vi "Replace Sub VI.vi"(8 "error in (no error)":errorcluster, 11 "VI in":refnum<vi>) -> (0 "error out":errorcluster, 3 "VI out":refnum<vi>)   [LabVIEW 2020, in "Responsive Mock Class Generator.lvclass"]
uses:
  Responsive Mock Class Generator.lvclass
  <vilib>/Utility/traverseref.llb/TRef TravTarget.ctl
  <vilib>/Utility/traverseref.llb/VI Scripting - Traverse.lvlib
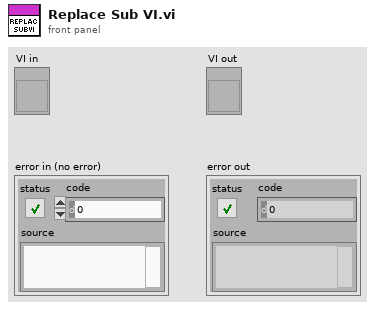
[diagram p1: front panel]
types:
  T1 = typedef "TRef TravTarget.ctl" = enum16{"FP", "BD", "Other"}
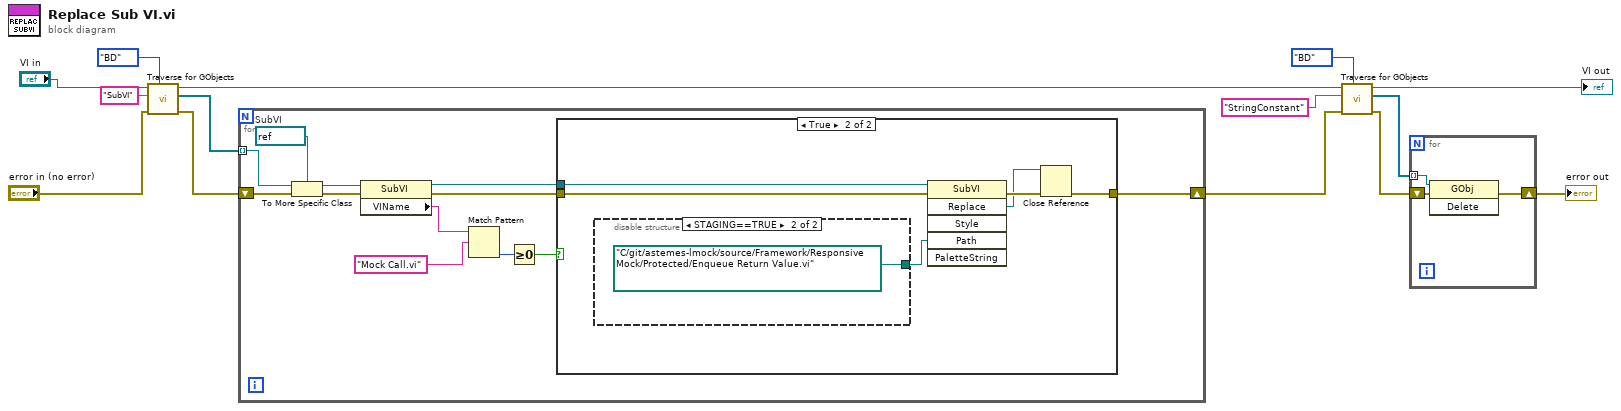
[diagram p0: block diagram]
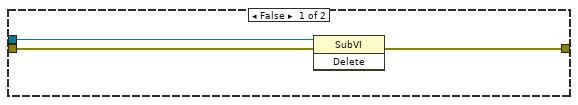
[diagram p2: hidden frame]
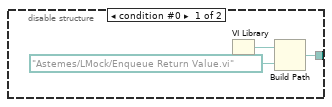
[diagram p3: hidden frame]
diagram:
  n1 = call <vilib>:"Traverse for GObjects.vi"("Traverse Target"=TRef_TravTarget."BD", "error in (no error)"="error in (no error)", "Class Name"="SubVI", "VI Refnum"="VI in") -> ("error out"=w9:errorcluster, "References"=w10:refnum<vi>[], "dup VI Refnum"=w8:refnum<vi>)  [unwired: 4 in, 1 out]
  n2 = for {
    tunnel: w10 -> [w22] mode=indexing
    shift-right: [w15] -> w3
    shift-left: w9 -> [w26]
    w20 = refnum<vi> refnum  # SubVI
    n3 = To More Specific Class(target class=w20, reference=w22, error in=w26) -> (specific class reference=w21:refnum<vi>, error out=w23:errorcluster)
    n4 = property class="SubVI"(reference=w21, error in=w23) -> (reference out=w24:refnum<vi>, error out=w25:errorcluster, "VIName"=w17:string)
    n5 = Match Pattern(string=w17, regular expression="Mock Call.vi") -> (offset past match=w19:i32)  [unwired: 1 in, 3 out]
    n6 = Greater Or Equal To 0?(x=w19) -> (x >= 0?=w18:bool)
    n7 = case shown="True" w18 {
      tunnel: [w27 w31] -> w15
      tunnel: w25 -> [w28 w33]
      tunnel: w24 -> [w29 w32]
      frame False {
        n8 = invoke class="SubVI" method="Delete"(reference=w29, error in=w28) -> (error out=w27:errorcluster)  [unwired: 1 in, 2 out]
      }
      frame True {
        n9 = disable-structure shown="STAGING==TRUE" {
          disable-tunnel: [w36 path "C:/git/astemes-lmock/source/Framework/Responsive Mock/Protected/Enqueue Return Value.vi" ("appended path")] -> w34
          frame condition #0 {
            n10 = VI Library() -> (path=w37:path)
            n11 = Build Path(base path=w37, name or relative path=path "Astemes/LMock/Enqueue Return Value.vi" ("class path")) -> (appended path=w36:path)
          }
          frame condition #1 (active) {
          }
        }
        n12 = invoke class="SubVI" method="Replace"(reference=w32, error in=w33, "Path"=w34) -> (error out=w35:errorcluster, "Replace"=w30:refnum<vi>)  [unwired: 3 in, 4 out]
        n13 = Close Reference(reference=w30, error in (no error)=w35) -> (error out=w31:errorcluster)
      }
    }
  }
  n14 = call <vilib>:"Traverse for GObjects.vi"("Traverse Target"=TRef_TravTarget."BD", "error in (no error)"=w3, "Class Name"="StringConstant", "VI Refnum"=w8) -> ("error out"=w2:errorcluster, "References"=w1:refnum<vi>[], "dup VI Refnum"=→"VI out":refnum<vi>)  [unwired: 4 in, 1 out]
  n15 = for {
    shift-right: [w41] -> w4
    shift-left: w2 -> [w42]
    tunnel: w1 -> [w40] mode=indexing
    n16 = invoke class="GObj" method="Delete"(reference=w40, error in=w42) -> (error out=w41:errorcluster)  [unwired: 1 in, 2 out]
  }
  "error out" <- w4
